vi "BioFeedback9(export8ChanelToMatlab+VR).vi"(0 "UI Data Right":path=path "C:/Users/Tinggroup/Desktop/VRMuscleActivationVisualizer/VRBiofeedback_v2/assets/RightEMGData.txt", 7 "Frames Per Second":dbl=30.0, 9 "Start Trial":bool, 11 "End Trial":bool, 12 "Data Directory":path, 13 "File Name":string, 14 "Extension":string="_EMG.txt") -> ()   [LabVIEW 2016]
uses:
  <vilib>/Utility/error.llb/DialogType.ctl
  <vilib>/Analysis/5stat.llb/RMS (DBL).vi
  <vilib>/Waveform/WDTOps.llb/WDT Append Waveforms DBL.vi
  <vilib>/Waveform/WDTFileIO.llb/Export Waveforms To Spreadsheet File (1D).vi
  <vilib>/Analysis/NI_AALPro.lvlib
panel:
  out "sampleRawWaveforms":waveform(dbl)[](array[waveform])
  out "rawWaveforms":waveform(dbl)[](array[waveform])
  in  "UI Ampl Error Path":path=path "C:/Users/Tinggroup/Desktop/VRMuscleActivationVisualizer/VRBiofeedback_v2/assets/BiofeedbackAmplitudeError.txt"
  in  "UI L/R Error Path":path=path "C:/Users/Tinggroup/Desktop/VRMuscleActivationVisualizer/VRBiofeedback_v2/assets/BiofeedbackLRError.txt"
  out "LeftPercentActivation":dbl
  out "RightPercentActivation":dbl
  out "LeftMovingAvg":dbl
  out "RightMovingAvg":dbl
  out "Stability Data":dbl[](array[numeric])
  in  "StabilityBufferFramesCount":dbl=1.0
  out "StabilityFramesCount":dbl
  in  "GuageStability":bool
  out "StdDev":dbl
  out "Mean":dbl
  out "Min":dbl
  out "Max":dbl
  in  "AutoAnalyzeStablity":bool
  out "RMS Left Single Bucket":dbl(graph)
  out "PointCluster":cluster{dbl[], dbl[]}
  out "combined y value":dbl
  out "Acquiring Max":bool
  in  "endGetMax":bool
  in  "startGetMax":bool
  in  "Right Max":dbl
  in  "Left Max":dbl
  in  "Amplitude Error":dbl
  in  "L/R error":dbl
  out "Target Graph":cluster{dbl[], dbl[]}[](graph)
  in  "RightSignalB":dbl=6.0
  in  "RightSignalA":dbl=5.0
  in  "LefftSignalB":dbl=2.0
  in  "LeftSignalA":dbl=1.0
  out "Aggregate 8":waveform(dbl)[](array[waveform])
  in  "UI Data Left":path=path "C:/Users/Tinggroup/Desktop/VRMuscleActivationVisualizer/VRBiofeedback_v2/assets/LeftEMGData.txt"
  in  "EMG Input Device\nProduct Type":string="USB-6009"
  out "DispLeftMovingAvg":dbl(slide) max=1.0 scale=0.0..100.0
  out "DispRightMovingAvg":dbl(slide) max=0.01 scale=0.0..100.0
  out "RMS Right":dbl(graph)
  out "RMS Left":dbl(graph)
  out "RMS 8":dbl(graph)
  out "RMS 7":dbl(graph)
  out "RMS 6":dbl(graph)
  out "RMS 5":dbl(graph)
  out "RMS 4":dbl(graph)
  out "RMS 3":dbl(graph)
  out "RMS 2":dbl(graph)
  out "RMS 1":dbl(graph)
  out "Aggregate7":waveform(dbl)[](array[waveform])
  out "Aggregate6":waveform(dbl)[](array[waveform])
  out "Aggregate5":waveform(dbl)[](array[waveform])
  out "Aggregate4":waveform(dbl)[](array[waveform])
  out "Aggregate3":waveform(dbl)[](array[waveform])
  out "Aggregate2":waveform(dbl)[](array[waveform])
  out "Aggregate1":waveform(dbl)[](array[waveform])
  out "Wfm8":waveform(dbl)(graph)
  out "Wfm7":waveform(dbl)(graph)
  out "Wfm6":waveform(dbl)(graph)
  out "Wfm5":waveform(dbl)(graph)
  out "Wfm4":waveform(dbl)(graph)
  out "Wfm3":waveform(dbl)(graph)
  out "Wfm2":waveform(dbl)(graph)
  out "Wfm1":waveform(dbl)(graph)
  out "Sample Raw Waveforms":waveform(dbl)[](graph)
  in  "UI Percent Path":path=path "C:/Users/Tinggroup/Desktop/VRMuscleActivationVisualizer/VRBiofeedback_v2/assets/BiofeedbackTargetPercentage.txt"
  in  "Target Percentage":dbl=10.0
  out "Trial In Progress":bool
  in  "Trial Number":dbl
  in  "MARK":bool
  in  "Lower Cut-Off":dbl=20.0
  in  "Upper Cut-Off":dbl=300.0
  out "raw data":dynamicdata(graph)
  out "Bufffer Index":dbl
  out "Frames in Buffer":dbl
  out "Samples per frame":dbl
  out "Reset Data Acquisition\nAnd UI Updating":bool=TRUE
  in  "Moving Average Length (s)":dbl=0.5
  in  "Sample rate (Hz)":dbl=2000.0
  in  "End Program":bool
  # "These \nSet \nThe \nTarget\nBox Size"
  # "Save Trial Data"
  # "These scale\nthe thermometers\nand are used in\nmean calculation"
  # "Auto Analyze Stability begins calculating stability\nAs soon as dot enters the target zone and stops \nonce the dot leaves the target zone"
  # "for testing smaller sample\nsizes in getting max/min\nand stability data"
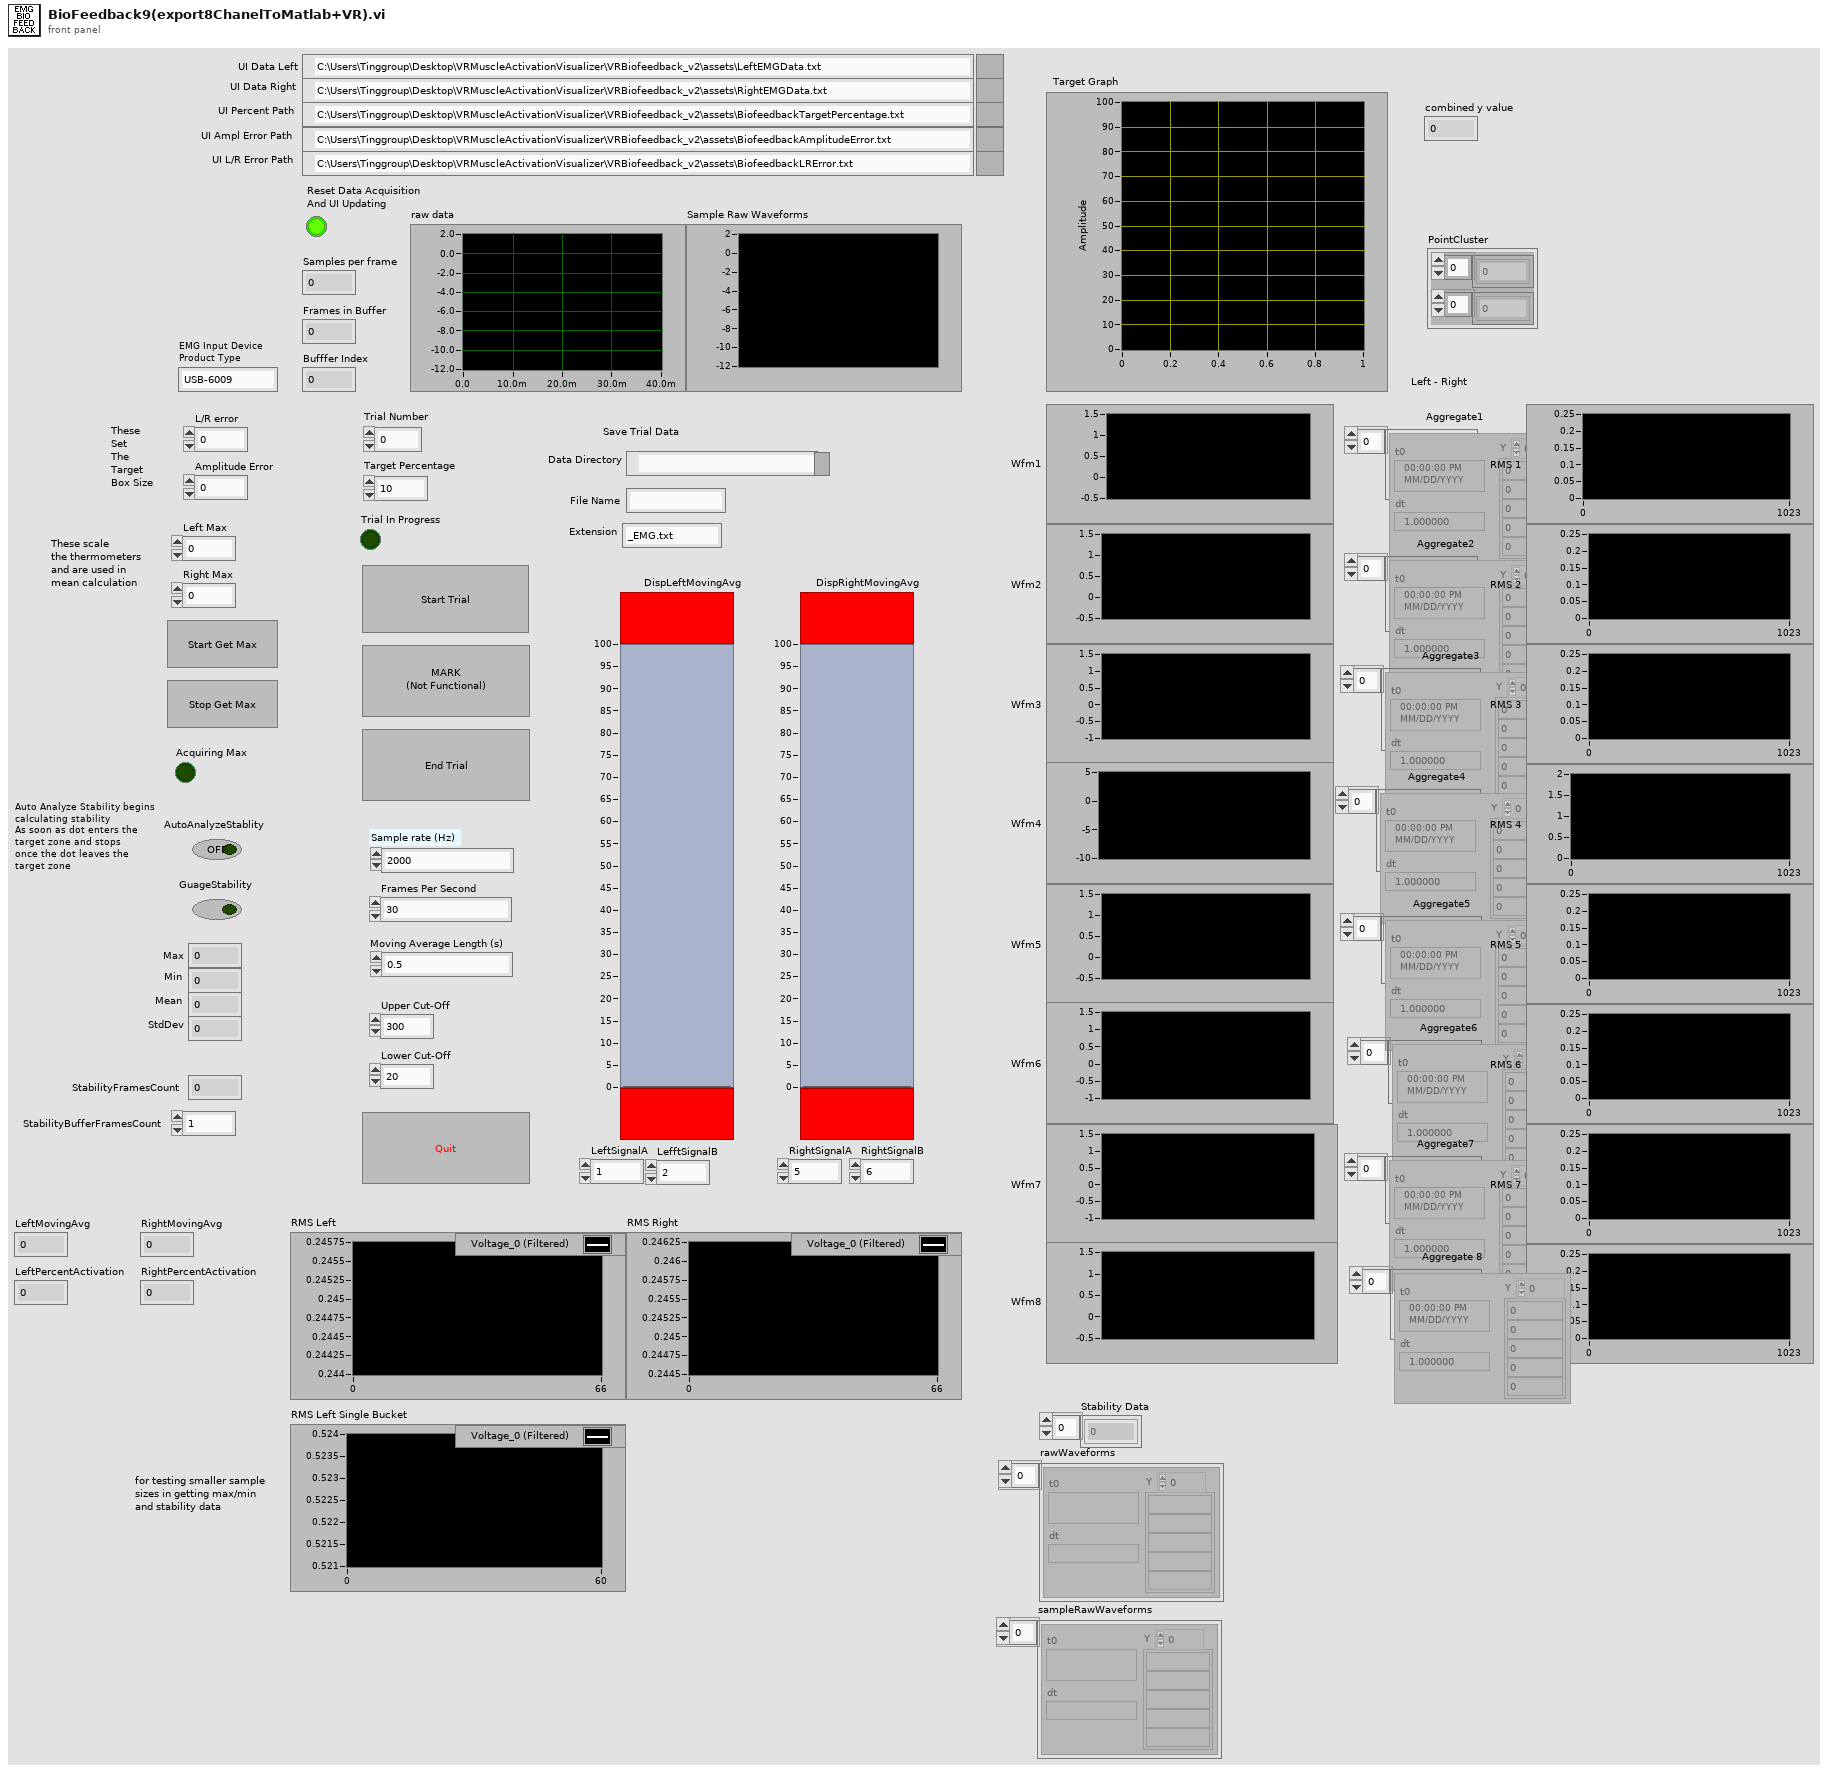
[diagram p1: front panel]
types:
  T1 = typedef "DialogType.ctl" = u16
  T2 = typedef "WaveformArrayControl.ctl" = waveform(dbl)[]
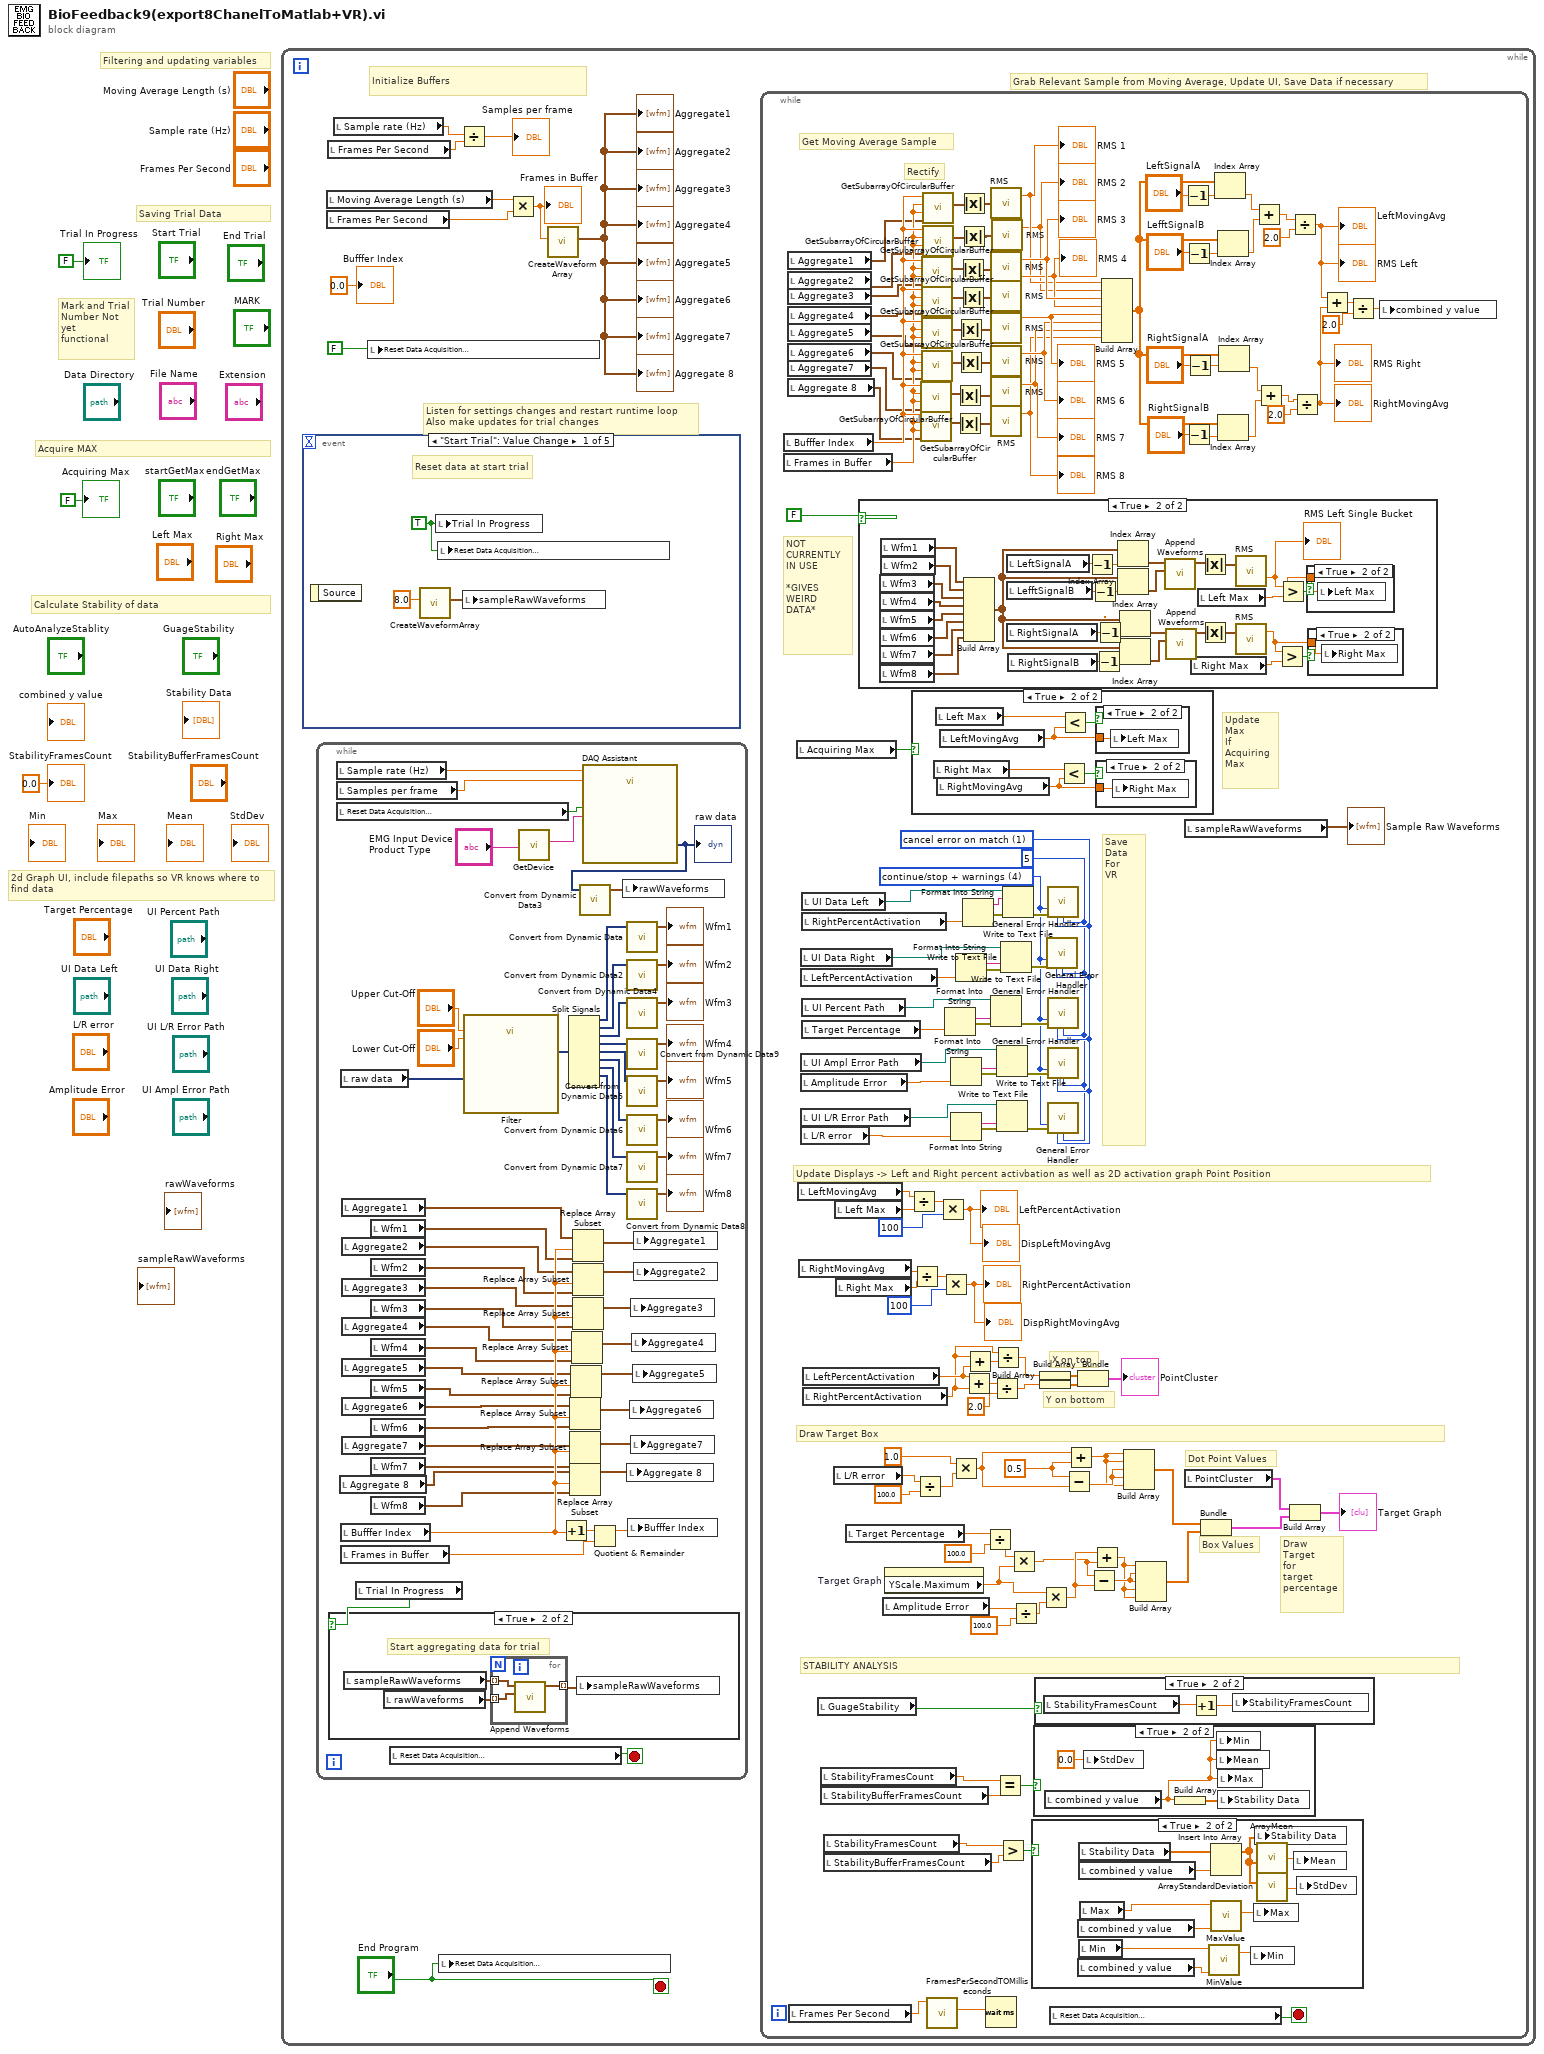
[diagram p0: block diagram]
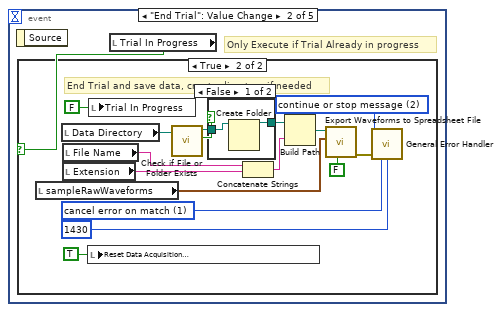
[diagram p2: hidden frame]
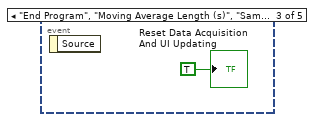
[diagram p5: hidden frame]
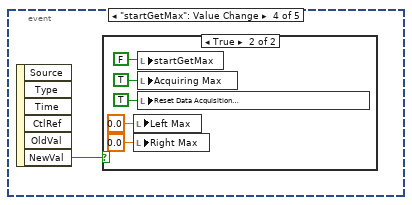
[diagram p6: hidden frame]
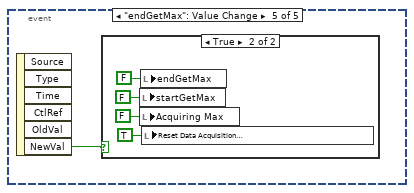
[diagram p8: hidden frame]
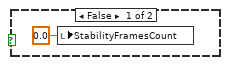
[diagram p12: hidden frame]
diagram:
  # "Calculate Stability of data"
  # "Acquire MAX"
  # "Filtering and updating variables"
  # "Saving Trial Data"
  # "2d Graph UI, include filepaths so VR knows where to find data"
  # "Mark and Trial Number Not yet \nfunctional"
  n1 = while {
    stop <- "End Program" stop-if-true
    # "Grab Relevant Sample from Moving Average, Update UI, Save Data if necessary"
    # "Initialize Buffers"
    # "Listen for settings changes and restart runtime loop\nAlso make updates for trial changes"
    n2 = event shown="[0] \"Start Trial\": Value Change" {
      selector: _ -> [_ _ _ _ _]
      dyn-events: _ -> [_ _ _ _ _]
      timeout: _ -> [_ _ _ _ _]
      event "Start Trial": Value Change {
        w16 = TRUE ("Trial In Progress")
        # "Reset data at start trial"
        n3 = event-data() -> ()  [unwired: 1 in, 1 out]
        n4 = call "CreateWaveformArray.vi"("bufferSize"=8.0) -> ("initialized array"=w15:waveform(dbl)[])  [unwired: 5 in, 1 out]
        n5 = local write "Trial In Progress"(w16) -> ()
        n6 = local write "Reset Data Acquisition\nAnd UI Updating"(w16) -> ()
        n7 = local write "sampleRawWaveforms"(w15) -> ()
      }
      event "End Trial": Value Change {
        # "Only Execute if Trial Already in progress"
        n8 = event-data() -> ()  [unwired: 1 in, 1 out]
        n9 = local read "Trial In Progress"() -> (w17:bool)
        n10 = case shown="True" w17 {
          frame False {
          }
          frame True {
            w26 = T1 2 items=["no dialog", "OK message", "continue or stop message", "OK message + warnings", "continue/stop + warnings"] ("type of dialog (OK msg:1)")
            w27 = 1 items=["no exception", "cancel error on match", "set error on match"] ("[exception action] (none:0)")
            # "End Trial and save data, create directory if needed"
            n11 = local read "sampleRawWaveforms"() -> (w19:waveform(dbl)[])
            n12 = local read "Data Directory"() -> (w29:path)
            n13 = local read "File Name"() -> (w21:string)
            n14 = local read "Extension"() -> (w22:string)
            n15 = local write "Reset Data Acquisition\nAnd UI Updating"(TRUE ("Reset Data Acquisition\nAnd UI Updating")) -> ()
            n16 = local write "Trial In Progress"(FALSE ("Trial In Progress")) -> ()
            n17 = call <vilib>:"Check if File or Folder Exists.vi"("path"=w29) -> ("file or folder exists?"=w31:bool, "dup path"=w30:path)  [unwired: 8 in, 1 out]
            n18 = case shown="False" w31 {
              tunnel: [w34 w36] -> w25
              tunnel: w30 -> [w35 w36]
              frame False {
                n19 = Create Folder(path (use dialog)=w35) -> (created path=w34:path)  [unwired: 2 in, 2 out]
              }
              frame True {
              }
            }
            n20 = Concatenate Strings(w21, w22) -> (w20:string)
            n21 = Build Path(base path=w25, name or relative path=w20) -> (appended path=w24:path)
            n22 = call-poly <vilib>:"Export Waveforms to Spreadsheet File.vi"("append to file? (new file:F)"=FALSE, "waveforms"=w19, "file path (dialog if empty)"=w24) -> ("error out"=w18:errorcluster)  [unwired: 7 in, 1 out]
            n23 = call <vilib>:"General Error Handler.vi"("type of dialog (OK msg:1)"=w26, "error in (no error)"=w18, "[exception action] (none:0)"=w27, "[exception code]"=1430) -> ()  [unwired: 7 in, 5 out]
          }
        }
      }
      event "End Program", "Moving Average Length (s)", "Sample rate (Hz)", "Frames Per Second": Value Change {
        n24 = event-data() -> ()  [unwired: 1 in, 1 out]
        "Reset Data Acquisition\nAnd UI Updating" <- TRUE
      }
      event "startGetMax": Value Change {
        n25 = event-data() -> ("NewVal"=w38:bool)  [unwired: 1 in, 5 out]
        n26 = case shown="True" w38 {
          frame False {
          }
          frame True {
            n27 = local write "Left Max"(0.0 ("Left Max")) -> ()
            n28 = local write "Right Max"(0.0 ("Right Max")) -> ()
            n29 = local write "startGetMax"(FALSE) -> ()
            n30 = local write "Acquiring Max"(TRUE ("Acquiring Max")) -> ()
            n31 = local write "Reset Data Acquisition\nAnd UI Updating"(TRUE ("Reset Data Acquisition\nAnd UI Updating")) -> ()
          }
        }
      }
      event "endGetMax": Value Change {
        n32 = event-data() -> ("NewVal"=w44:bool)  [unwired: 1 in, 5 out]
        n33 = case shown="True" w44 {
          frame False {
          }
          frame True {
            n34 = local write "startGetMax"(FALSE ("startGetMax")) -> ()
            n35 = local write "Acquiring Max"(FALSE ("Acquiring Max")) -> ()
            n36 = local write "endGetMax"(FALSE ("endGetMax")) -> ()
            n37 = local write "Reset Data Acquisition\nAnd UI Updating"(TRUE ("Reset Data Acquisition\nAnd UI Updating")) -> ()
          }
        }
      }
    }
    n38 = while {
      stop <- w297 stop-if-true
      n39 = local read "Sample rate (Hz)"() -> (w304:dbl)
      n40 = local read "Samples per frame"() -> (w303:dbl)
      n41 = local read "Reset Data Acquisition\nAnd UI Updating"() -> (w296:bool)
      n42 = local read "Aggregate 8"() -> (w252:waveform(dbl)[])
      n43 = local read "raw data"() -> (w302:dynamicdata)
      n44 = local read "Bufffer Index"() -> (w277:dbl)
      n45 = local read "Frames in Buffer"() -> (w299:dbl)
      n46 = local read "Aggregate1"() -> (w276:waveform(dbl)[])
      n47 = local read "Aggregate2"() -> (w274:waveform(dbl)[])
      n48 = local read "Aggregate3"() -> (w272:waveform(dbl)[])
      n49 = local read "Aggregate4"() -> (w270:waveform(dbl)[])
      n50 = local read "Aggregate5"() -> (w268:waveform(dbl)[])
      n51 = local read "Aggregate6"() -> (w266:waveform(dbl)[])
      n52 = local read "Aggregate7"() -> (w264:waveform(dbl)[])
      n53 = local read "Trial In Progress"() -> (w254:bool)
      n54 = case shown="True" w254 {
        frame False {
        }
        frame True {
          # "Start aggregating data for trial"
          n55 = local read "sampleRawWaveforms"() -> (w306:waveform(dbl)[])
          n56 = local read "rawWaveforms"() -> (w307:waveform(dbl)[])
          n57 = for {
            tunnel: w307 -> [w309] mode=indexing
            tunnel: w306 -> [w310] mode=indexing
            tunnel: [w308] -> w305 mode=indexing
            n58 = call-poly <vilib>:"Append Waveforms.vi"("waveform B"=w309, "waveform A"=w310) -> ("waveform out"=w308:waveform(dbl))  [unwired: 8 in, 1 out]
          }
          n59 = local write "sampleRawWaveforms"(w305) -> ()
        }
      }
      n60 = local read "Wfm1"() -> (w275:waveform(dbl))
      n61 = local read "Wfm2"() -> (w273:waveform(dbl))
      n62 = local read "Wfm3"() -> (w271:waveform(dbl))
      n63 = local read "Wfm4"() -> (w269:waveform(dbl))
      n64 = local read "Wfm5"() -> (w267:waveform(dbl))
      n65 = local read "Wfm6"() -> (w265:waveform(dbl))
      n66 = local read "Wfm7"() -> (w263:waveform(dbl))
      n67 = local read "Wfm8"() -> (w262:waveform(dbl))
      n68 = local read "Reset Data Acquisition\nAnd UI Updating"() -> (w297:bool)
      n69 = call "Filter"("Lower Cut-Off"="Lower Cut-Off", "Upper Cut-Off"="Upper Cut-Off", "Signal"=w302) -> ("Filtered Signal"=w294:dynamicdata)  [unwired: 7 in, 1 out]
      n70 = call "GetDevice.vi"("EMG Input Device\nProduct Type"="EMG Input Device\nProduct Type") -> ("DAQmx Device Name"=w250:tag)  [unwired: 10 in]
      n71 = Increment(x=w277) -> (x+1=w298:dbl)
      n72 = Split Signals(w294) -> (w293:dynamicdata, w292:dynamicdata, w291:dynamicdata, w290:dynamicdata, w289:dynamicdata, w288:dynamicdata, w287:dynamicdata, w286:dynamicdata)  [unwired: 9 in, 1 out]
      n73 = Replace Array Subset(array=w266, new element=w265, index=w277) -> (w256:waveform(dbl)[])
      n74 = Replace Array Subset(array=w264, new element=w263, index=w277) -> (w255:waveform(dbl)[])
      n75 = Replace Array Subset(array=w252, new element=w262, index=w277) -> (w253:waveform(dbl)[])
      n76 = Replace Array Subset(array=w268, new element=w267, index=w277) -> (w257:waveform(dbl)[])
      n77 = Replace Array Subset(array=w270, new element=w269, index=w277) -> (w258:waveform(dbl)[])
      n78 = Replace Array Subset(array=w276, new element=w275, index=w277) -> (w261:waveform(dbl)[])
      n79 = Replace Array Subset(array=w274, new element=w273, index=w277) -> (w260:waveform(dbl)[])
      n80 = Replace Array Subset(array=w272, new element=w271, index=w277) -> (w259:waveform(dbl)[])
      n81 = call "DAQ Assistant"("rate"=w304, "number of samples"=w303, "stop (T)"=w296, "device name"=w250) -> ("data"=w249:dynamicdata)  [unwired: 13 in, 2 out]
      "raw data" <- w249
      n82 = call "Convert from Dynamic Data3"("Dynamic Data Type"=w249) -> ("Array of Waveform"=w248:waveform(dbl)[])  [unwired: 3 in]
      n83 = Quotient & Remainder(x=w298, y=w299) -> (x-y*floor(x/y)=w300:dbl)  [unwired: 1 out]
      n84 = local write "rawWaveforms"(w248) -> ()
      n85 = call "Convert from Dynamic Data"("Dynamic Data Type"=w293) -> ("Waveform"=→"Wfm1":waveform(dbl))  [unwired: 3 in]
      n86 = call "Convert from Dynamic Data2"("Dynamic Data Type"=w292) -> ("Waveform"=→"Wfm2":waveform(dbl))  [unwired: 3 in]
      n87 = call "Convert from Dynamic Data4"("Dynamic Data Type"=w291) -> ("Waveform"=→"Wfm3":waveform(dbl))  [unwired: 3 in]
      n88 = call "Convert from Dynamic Data9"("Dynamic Data Type"=w290) -> ("Waveform"=→"Wfm4":waveform(dbl))  [unwired: 3 in]
      n89 = call "Convert from Dynamic Data5"("Dynamic Data Type"=w289) -> ("Waveform"=→"Wfm5":waveform(dbl))  [unwired: 3 in]
      n90 = call "Convert from Dynamic Data6"("Dynamic Data Type"=w288) -> ("Waveform"=→"Wfm6":waveform(dbl))  [unwired: 3 in]
      n91 = call "Convert from Dynamic Data7"("Dynamic Data Type"=w287) -> ("Waveform"=→"Wfm7":waveform(dbl))  [unwired: 3 in]
      n92 = call "Convert from Dynamic Data8"("Dynamic Data Type"=w286) -> ("Waveform"=→"Wfm8":waveform(dbl))  [unwired: 3 in]
      n93 = local write "Aggregate 8"(w253) -> ()
      n94 = local write "Bufffer Index"(w300) -> ()
      n95 = local write "Aggregate6"(w256) -> ()
      n96 = local write "Aggregate3"(w259) -> ()
      n97 = local write "Aggregate7"(w255) -> ()
      n98 = local write "Aggregate4"(w258) -> ()
      n99 = local write "Aggregate5"(w257) -> ()
      n100 = local write "Aggregate1"(w261) -> ()
      n101 = local write "Aggregate2"(w260) -> ()
    }
    n102 = local read "Moving Average Length (s)"() -> (w10:dbl)
    n103 = local read "Frames Per Second"() -> (w9:dbl)
    n104 = local read "Frames Per Second"() -> (w12:dbl)
    n105 = local read "Sample rate (Hz)"() -> (w13:dbl)
    n106 = local write "Reset Data Acquisition\nAnd UI Updating"(FALSE) -> ()
    n107 = local write "Reset Data Acquisition\nAnd UI Updating"("End Program") -> ()
    n108 = Divide(x=w13, y=w12) -> (x/y=→"Samples per frame":dbl)
    n109 = Multiply(x=w10, y=w9) -> (x*y=w6:dbl)
    "Frames in Buffer" <- w6
    n110 = call "CreateWaveformArray.vi"("bufferSize"=w6) -> ("initialized array"=→"Aggregate1" →"Aggregate2" →"Aggregate3" →"Aggregate4" →"Aggregate5" →"Aggregate6" →"Aggregate7" →"Aggregate 8":waveform(dbl)[])  [unwired: 5 in, 1 out]
    n111 = while {
      stop <- w189 stop-if-true
      w107 = 0.5 ("element")
      w51 = T1 4 items=["no dialog", "OK message", "continue or stop message", "OK message + warnings", "continue/stop + warnings"] ("type of dialog (OK msg:1)")
      w50 = 1 items=["no exception", "cancel error on match", "set error on match"] ("[exception action] (none:0)")
      w49 = 5 ("[exception code]")
      # "Y on bottom"
      # "X on top"
      # "Dot Point Values"
      # "Box Values"
      # "Update Displays -> Left and Right percent activbation as well as 2D activation graph Point Position"
      # "STABILITY ANALYSIS"
      # "NOT\nCURRENTLY\nIN USE\n\n*GIVES\nWEIRD\nDATA*"
      # "Draw \nTarget\nfor\ntarget\npercentage"
      # "Draw Target Box"
      # "Update\nMax\nIf \nAcquiring\nMax"
      # "Save\nData\nFor\nVR"
      # "Get Moving Average Sample"
      # "Rectify"
      n112 = local read "Bufffer Index"() -> (w180:dbl)
      n113 = local read "Frames in Buffer"() -> (w179:dbl)
      n114 = local read "Aggregate1"() -> (w178:waveform(dbl)[])
      n115 = local read "Aggregate2"() -> (w174:waveform(dbl)[])
      n116 = local read "Aggregate3"() -> (w177:waveform(dbl)[])
      n117 = local read "Aggregate4"() -> (w173:waveform(dbl)[])
      n118 = local read "Aggregate5"() -> (w176:waveform(dbl)[])
      n119 = local read "Aggregate6"() -> (w175:waveform(dbl)[])
      n120 = local read "Aggregate7"() -> (w172:waveform(dbl)[])
      n121 = local read "Aggregate 8"() -> (w146:waveform(dbl)[])
      n122 = local read "Frames Per Second"() -> (w188:dbl)
      n123 = local read "Acquiring Max"() -> (w91:bool)
      n124 = local read "LeftMovingAvg"() -> (w80:dbl)
      n125 = local read "RightMovingAvg"() -> (w76:dbl)
      n126 = local read "UI Data Right"() -> (w184:path)
      n127 = local read "LeftPercentActivation"() -> (w182:dbl)
      n128 = local read "UI Ampl Error Path"() -> (w52:path)
      n129 = local read "Amplitude Error"() -> (w53:dbl)
      n130 = local read "UI L/R Error Path"() -> (w55:path)
      n131 = local read "L/R error"() -> (w54:dbl)
      n132 = local read "UI Data Left"() -> (w154:path)
      n133 = local read "RightPercentActivation"() -> (w156:dbl)
      n134 = local read "UI Percent Path"() -> (w148:path)
      n135 = local read "Target Percentage"() -> (w147:dbl)
      n136 = local read "LeftPercentActivation"() -> (w69:dbl)
      n137 = local read "RightPercentActivation"() -> (w67:dbl)
      n138 = local read "GuageStability"() -> (w89:bool)
      n139 = local read "StabilityFramesCount"() -> (w88:dbl)
      n140 = local read "StabilityBufferFramesCount"() -> (w87:dbl)
      n141 = local read "StabilityFramesCount"() -> (w85:dbl)
      n142 = local read "StabilityBufferFramesCount"() -> (w84:dbl)
      n143 = local read "L/R error"() -> (w126:dbl)
      n144 = local read "Left Max"() -> (w79:dbl)
      n145 = local read "Right Max"() -> (w75:dbl)
      n146 = local read "Target Percentage"() -> (w123:dbl)
      n147 = case shown="True" FALSE {
        frame False {
        }
        frame True {
          n148 = local read "Wfm3"() -> (w238:waveform(dbl))
          n149 = local read "Wfm4"() -> (w237:waveform(dbl))
          n150 = local read "Wfm5"() -> (w241:waveform(dbl))
          n151 = local read "Wfm6"() -> (w242:waveform(dbl))
          n152 = local read "Wfm7"() -> (w243:waveform(dbl))
          n153 = local read "Wfm8"() -> (w244:waveform(dbl))
          n154 = local read "Wfm1"() -> (w240:waveform(dbl))
          n155 = local read "Wfm2"() -> (w239:waveform(dbl))
          n156 = Build Array(w240, w239, w238, w237, w241, w242, w243, w244) -> (w236:waveform(dbl)[])
          n157 = local read "LeftSignalA"() -> (w222:dbl)
          n158 = local read "LefftSignalB"() -> (w220:dbl)
          n159 = local read "RightSignalA"() -> (w218:dbl)
          n160 = local read "RightSignalB"() -> (w215:dbl)
          n161 = Decrement(x=w222) -> (x-1=w221:dbl)
          n162 = Decrement(x=w220) -> (x-1=w219:dbl)
          n163 = Decrement(x=w215) -> (x-1=w216:dbl)
          n164 = Decrement(x=w218) -> (x-1=w217:dbl)
          n165 = Index Array(array=w236, index=w221) -> (element=w223:waveform(dbl))
          n166 = Index Array(array=w236, index=w219) -> (element=w224:waveform(dbl))
          n167 = Index Array(array=w236, index=w217) -> (element=w235:waveform(dbl))
          n168 = Index Array(array=w236, index=w216) -> (element=w234:waveform(dbl))
          n169 = call-poly <vilib>:"Append Waveforms.vi"("waveform B"=w224, "waveform A"=w223) -> ("waveform out"=w230:waveform(dbl))  [unwired: 8 in, 1 out]
          n170 = call-poly <vilib>:"Append Waveforms.vi"("waveform B"=w234, "waveform A"=w235) -> ("waveform out"=w233:waveform(dbl))  [unwired: 8 in, 1 out]
          n171 = local read "Right Max"() -> (w229:dbl)
          n172 = local read "Left Max"() -> (w245:dbl)
          n173 = Absolute Value(x=w230) -> (abs(x)=w231:waveform(dbl))
          n174 = Absolute Value(x=w233) -> (abs(x)=w232:waveform(dbl))
          n175 = call-poly <vilib>:"RMS.vi"("X"=w231) -> ("rms value"=w225:dbl)  [unwired: 1 out]
          "RMS Left Single Bucket" <- w225
          n176 = call-poly <vilib>:"RMS.vi"("X"=w232) -> ("rms value"=w228:dbl)  [unwired: 1 out]
          n177 = Greater?(x=w228, y=w229) -> (0:w227:bool)
          n178 = Greater?(x=w225, y=w245) -> (0:w226:bool)
          n179 = case shown="True" w226 {
            tunnel: w225 -> [_ w247]
            frame False {
            }
            frame True {
              n180 = local write "Left Max"(w247) -> ()
            }
          }
          n181 = case shown="True" w227 {
            tunnel: w228 -> [_ w246]
            frame False {
            }
            frame True {
              n182 = local write "Right Max"(w246) -> ()
            }
          }
        }
      }
      n183 = local read "Amplitude Error"() -> (w125:dbl)
      n184 = property on="Target Graph" class="XYGraph (strict)"() -> ("YScale.Maximum"=w105:dbl)  [unwired: 2 in, 2 out]
      n185 = Divide(x=w80, y=w79) -> (x/y=w81:dbl)
      n186 = case shown="True" w91 {
        frame False {
        }
        frame True {
          n187 = local read "Right Max"() -> (w209:dbl)
          n188 = local read "Left Max"() -> (w212:dbl)
          n189 = local read "RightMovingAvg"() -> (w207:dbl)
          n190 = local read "LeftMovingAvg"() -> (w211:dbl)
          n191 = Less?(x=w209, y=w207) -> (x < y?=w208:bool)
          n192 = Less?(x=w212, y=w211) -> (x < y?=w210:bool)
          n193 = case shown="True" w210 {
            tunnel: w211 -> [_ w214]
            frame False {
            }
            frame True {
              n194 = local write "Left Max"(w214) -> ()
            }
          }
          n195 = case shown="True" w208 {
            tunnel: w207 -> [_ w213]
            frame False {
            }
            frame True {
              n196 = local write "Right Max"(w213) -> ()
            }
          }
        }
      }
      n197 = Divide(x=w76, y=w75) -> (x/y=w77:dbl)
      n198 = Divide(x=w126, y=100.0) -> (x/y=w115:dbl)
      n199 = call "GetSubarrayOfCircularBuffer.vi"("initialized array"=w172, "buffer size"=w179, "subset size"=w179, "start index"=w180) -> ("initialized array 2"=w165:T2)  [unwired: 7 in]
      n200 = call "GetSubarrayOfCircularBuffer.vi"("initialized array"=w146, "buffer size"=w179, "subset size"=w179, "start index"=w180) -> ("initialized array 2"=w164:T2)  [unwired: 7 in]
      n201 = call "GetSubarrayOfCircularBuffer.vi"("initialized array"=w177, "buffer size"=w179, "subset size"=w179, "start index"=w180) -> ("initialized array 2"=w169:T2)  [unwired: 7 in]
      n202 = call "GetSubarrayOfCircularBuffer.vi"("initialized array"=w173, "buffer size"=w179, "subset size"=w179, "start index"=w180) -> ("initialized array 2"=w168:T2)  [unwired: 7 in]
      n203 = call "GetSubarrayOfCircularBuffer.vi"("initialized array"=w176, "buffer size"=w179, "subset size"=w179, "start index"=w180) -> ("initialized array 2"=w167:T2)  [unwired: 7 in]
      n204 = call "GetSubarrayOfCircularBuffer.vi"("initialized array"=w175, "buffer size"=w179, "subset size"=w179, "start index"=w180) -> ("initialized array 2"=w166:T2)  [unwired: 7 in]
      n205 = call "GetSubarrayOfCircularBuffer.vi"("initialized array"=w178, "buffer size"=w179, "subset size"=w179, "start index"=w180) -> ("initialized array 2"=w171:T2)  [unwired: 7 in]
      n206 = call "GetSubarrayOfCircularBuffer.vi"("initialized array"=w174, "buffer size"=w179, "subset size"=w179, "start index"=w180) -> ("initialized array 2"=w170:T2)  [unwired: 7 in]
      n207 = call "FramesPerSecondTOMilliseconds.vi"("Thermometer\nFps"=w188) -> ("x*y"=w187:dbl)  [unwired: 10 in]
      n208 = Multiply(x=w81, y=100) -> (x*y=→"DispLeftMovingAvg" →"LeftPercentActivation":dbl)
      n209 = Multiply(x=w77, y=100) -> (x*y=→"DispRightMovingAvg" →"RightPercentActivation":dbl)
      n210 = Format Into String(w147) -> (resulting string=w149:string, error out=w150:errorcluster)  [unwired: 3 in]
      n211 = Format Into String(w53) -> (resulting string=w59:string, error out=w60:errorcluster)  [unwired: 3 in]
      n212 = Format Into String(w54) -> (resulting string=w56:string, error out=w57:errorcluster)  [unwired: 3 in]
      n213 = Multiply(x=1.0, y=w115) -> (x*y=w114:dbl)
      n214 = Absolute Value(x=w165) -> (abs(x)=w158:T2)
      n215 = Absolute Value(x=w164) -> (abs(x)=w157:T2)
      n216 = Absolute Value(x=w167) -> (abs(x)=w160:T2)
      n217 = Absolute Value(x=w166) -> (abs(x)=w159:T2)
      n218 = Format Into String(w182) -> (resulting string=w183:string, error out=w185:errorcluster)  [unwired: 3 in]
      n219 = Absolute Value(x=w169) -> (abs(x)=w162:T2)
      n220 = Absolute Value(x=w168) -> (abs(x)=w161:T2)
      n221 = Absolute Value(x=w171) -> (abs(x)=w163:T2)
      n222 = Absolute Value(x=w170) -> (abs(x)=w145:T2)
      n223 = Format Into String(w156) -> (resulting string=w153:string, error out=w155:errorcluster)  [unwired: 3 in]
      n224 = Add(x=w69, y=w67) -> (x+y=w71:dbl)
      n225 = Add(x=w67, y=w69) -> (x+y=w68:dbl)
      n226 = Divide(x=w123, y=100.0) -> (x/y=w106:dbl)
      n227 = Wait (ms)(milliseconds to wait=w187) -> ()  [unwired: 1 out]
      n228 = call-poly <vilib>:"RMS.vi"("X"=w163) -> ("rms value"=w139:dbl)  [unwired: 1 out]
      "RMS 1" <- w139
      n229 = call-poly <vilib>:"RMS.vi"("X"=w162) -> ("rms value"=w144:dbl)  [unwired: 1 out]
      "RMS 3" <- w144
      n230 = call-poly <vilib>:"RMS.vi"("X"=w161) -> ("rms value"=w143:dbl)  [unwired: 1 out]
      "RMS 4" <- w143
      n231 = call-poly <vilib>:"RMS.vi"("X"=w160) -> ("rms value"=w142:dbl)  [unwired: 1 out]
      "RMS 5" <- w142
      n232 = call-poly <vilib>:"RMS.vi"("X"=w159) -> ("rms value"=w141:dbl)  [unwired: 1 out]
      "RMS 6" <- w141
      n233 = call-poly <vilib>:"RMS.vi"("X"=w158) -> ("rms value"=w140:dbl)  [unwired: 1 out]
      "RMS 7" <- w140
      n234 = call-poly <vilib>:"RMS.vi"("X"=w157) -> ("rms value"=w137:dbl)  [unwired: 1 out]
      "RMS 8" <- w137
      n235 = Write to Text File(file (use dialog)=w148, text=w149, error in=w150) -> (error out=w151:errorcluster)  [unwired: 1 in, 2 out]
      n236 = call-poly <vilib>:"RMS.vi"("X"=w145) -> ("rms value"=w138:dbl)  [unwired: 1 out]
      "RMS 2" <- w138
      n237 = Divide(x=w71, y=2.0) -> (x/y=w70:dbl)
      n238 = Divide(x=w67, y=w68) -> (x/y=w66:dbl)
      n239 = Equal?(x=w88, y=w87) -> (x = y?=w86:bool)
      n240 = Write to Text File(file (use dialog)=w52, text=w59, error in=w60) -> (error out=w61:errorcluster)  [unwired: 1 in, 2 out]
      n241 = Write to Text File(file (use dialog)=w55, text=w56, error in=w57) -> (error out=w58:errorcluster)  [unwired: 1 in, 2 out]
      n242 = Greater?(x=w85, y=w84) -> (0:w83:bool)
      n243 = Write to Text File(file (use dialog)=w184, text=w183, error in=w185) -> (error out=w186:errorcluster)  [unwired: 1 in, 2 out]
      n244 = Write to Text File(file (use dialog)=w154, text=w153, error in=w155) -> (error out=w152:errorcluster)  [unwired: 1 in, 2 out]
      n245 = Multiply(x=w106, y=w105) -> (x*y=w111:dbl)
      n246 = Divide(x=w125, y=100.0) -> (x/y=w113:dbl)
      n247 = case shown="True" w83 {
        frame False {
        }
        frame True {
          n248 = local read "combined y value"() -> (w198:dbl)
          n249 = local read "combined y value"() -> (w195:dbl)
          n250 = local read "Stability Data"() -> (w200:dbl[])
          n251 = local read "combined y value"() -> (w199:dbl)
          n252 = local read "Min"() -> (w196:dbl)
          n253 = local read "Max"() -> (w197:dbl)
          n254 = call "MinValue.vi"("CurrentMin"=w196, "NewValue"=w195) -> ("Min"=w194:dbl)  [unwired: 8 in]
          n255 = Insert Into Array(array=w200, new element=w199) -> (w190:dbl[])  [unwired: 1 in]
          n256 = call "MaxValue.vi"("NewValue"=w198, "CurrentMax"=w197) -> ("Max"=w193:dbl)  [unwired: 9 in]
          n257 = local write "Min"(w194) -> ()
          n258 = local write "Max"(w193) -> ()
          n259 = local write "Stability Data"(w190) -> ()
          n260 = call "ArrayMean.vi"("Array"=w190) -> ("Mean"=w192:dbl)  [unwired: 10 in]
          n261 = call "ArrayStandardDeviation.vi"("Array"=w190) -> ("StdDev"=w191:dbl)  [unwired: 10 in]
          n262 = local write "Mean"(w192) -> ()
          n263 = local write "StdDev"(w191) -> ()
        }
      }
      n264 = case shown="True" w86 {
        frame False {
        }
        frame True {
          n265 = local read "combined y value"() -> (w201:dbl)
          n266 = local write "StdDev"(0.0 ("StdDev")) -> ()
          n267 = Build Array(w201) -> (w202:dbl[])
          n268 = local write "Min"(w201) -> ()
          n269 = local write "Mean"(w201) -> ()
          n270 = local write "Max"(w201) -> ()
          n271 = local write "Stability Data"(w202) -> ()
        }
      }
      n272 = case shown="True" w89 {
        frame False {
          n273 = local write "StabilityFramesCount"(0.0 ("StabilityFramescount")) -> ()
        }
        frame True {
          n274 = local read "StabilityFramesCount"() -> (w206:dbl)
          n275 = Increment(x=w206) -> (x+1=w205:dbl)
          n276 = local write "StabilityFramesCount"(w205) -> ()
        }
      }
      n277 = Build Array(w66) -> (w131:dbl[])
      n278 = Build Array(w70) -> (w129:dbl[])
      n279 = Multiply(x=w105, y=w113) -> (x*y=w112:dbl)
      n280 = call <vilib>:"General Error Handler.vi"("type of dialog (OK msg:1)"=w51, "error in (no error)"=w186, "[exception action] (none:0)"=w50, "[exception code]"=w49) -> ()  [unwired: 7 in, 5 out]
      n281 = call <vilib>:"General Error Handler.vi"("type of dialog (OK msg:1)"=w51, "error in (no error)"=w152, "[exception action] (none:0)"=w50, "[exception code]"=w49) -> ()  [unwired: 7 in, 5 out]
      n282 = call <vilib>:"General Error Handler.vi"("type of dialog (OK msg:1)"=w51, "error in (no error)"=w151, "[exception action] (none:0)"=w50, "[exception code]"=w49) -> ()  [unwired: 7 in, 5 out]
      n283 = call <vilib>:"General Error Handler.vi"("type of dialog (OK msg:1)"=w51, "error in (no error)"=w61, "[exception action] (none:0)"=w50, "[exception code]"=w49) -> ()  [unwired: 7 in, 5 out]
      n284 = call <vilib>:"General Error Handler.vi"("type of dialog (OK msg:1)"=w51, "error in (no error)"=w58, "[exception action] (none:0)"=w50, "[exception code]"=w49) -> ()  [unwired: 7 in, 5 out]
      n285 = local read "Reset Data Acquisition\nAnd UI Updating"() -> (w189:bool)
      n286 = Subtract(x=w107, y=w114) -> (x-y=w121:dbl)
      n287 = Add(x=w114, y=w107) -> (x+y=w116:dbl)
      n288 = Bundle(w131, w129) -> (→"PointCluster":cluster{dbl[], dbl[]})  [unwired: 1 in]
      n289 = Subtract(x=w111, y=w112) -> (x-y=w118:dbl)
      n290 = Add(x=w112, y=w111) -> (x+y=w117:dbl)
      n291 = Build Array(w139, w138, w144, w143, w142, w141, w140, w137) -> (w136:dbl[])
      n292 = Build Array(w116, w116, w121, w121, w116) -> (w109:dbl[])
      n293 = Build Array(w117, w118, w118, w117, w117) -> (w110:dbl[])
      n294 = Decrement(x="LeftSignalA") -> (x-1=w96:dbl)
      n295 = Decrement(x="LefftSignalB") -> (x-1=w98:dbl)
      n296 = Decrement(x="RightSignalB") -> (x-1=w94:dbl)
      n297 = Decrement(x="RightSignalA") -> (x-1=w92:dbl)
      n298 = local read "sampleRawWaveforms"() -> (→"Sample Raw Waveforms":waveform(dbl)[])
      n299 = local read "PointCluster"() -> (w104:cluster{dbl[], dbl[]})
      n300 = Bundle(w109, w110) -> (w119:cluster{dbl[], dbl[]})  [unwired: 1 in]
      n301 = Index Array(array=w136, index=w96) -> (element=w103:dbl)
      n302 = Index Array(array=w136, index=w98) -> (element=w102:dbl)
      n303 = Index Array(array=w136, index=w94) -> (element=w134:dbl)
      n304 = Index Array(array=w136, index=w92) -> (element=w135:dbl)
      n305 = Add(x=w103, y=w102) -> (x+y=w101:dbl)
      n306 = Add(x=w135, y=w134) -> (x+y=w132:dbl)
      n307 = Divide(x=w101, y=2.0) -> (x/y=w62:dbl)
      "RMS Left" <- w62
      "LeftMovingAvg" <- w62
      n308 = Build Array(w104, w119) -> (→"Target Graph":cluster{dbl[], dbl[]}[])
      n309 = Divide(x=w132, y=2.0) -> (x/y=w63:dbl)
      "RMS Right" <- w63
      "RightMovingAvg" <- w63
      n310 = Add(x=w62, y=w63) -> (x+y=w130:dbl)
      n311 = Divide(x=w130, y=2.0) -> (x/y=w128:dbl)
      n312 = local write "combined y value"(w128) -> ()
    }
    "Bufffer Index" <- 0.0 ("Bufffer Index")
  }
  "Trial In Progress" <- FALSE ("Trial In Progress")
  "Acquiring Max" <- FALSE ("Acquiring Max")
  "StabilityFramesCount" <- 0.0 ("StabilityFramescount")
